vi "gxml_BldTypeAttr.vi"(4 "error out":errorcluster, 5 "Variant":variant) -> (1 "error IO":errorcluster, 2 "TypeString":string)   [LabVIEW 2011, in "Third Party VIs.lvlib" / "GXML.lvlib"]
uses:
  GXML.lvlib
  <vilib>/Utility/VariantDataType/VariantType.lvlib
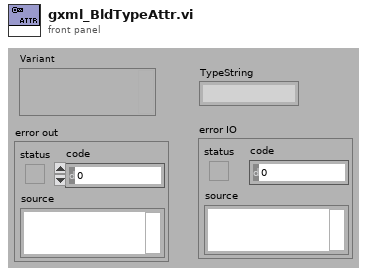
[diagram p1: front panel]
types:
  T1 = typedef "VariantType.lvlib/Type.ctl" = enum8{"Invalid Type", "Void", "I8", "I16", "I32", "I64", "U8", "U16", "U32", "U64", "Single Float", "Double Float", "Extended Float", "Single Complex", "Double Complex", "Extended Complex", "Enum U8", "Enum U16", "Enum U32", "Enum U64", "Single Float With Unit", "Double Float With Unit", "Extended Float With Unit", "Single Complex with Unit", "Double Complex with Unit", "Extended Complex with Unit", "Boolean", "String", "Path", "Picture", "Tag", "Array", "Cluster", "Variant", "LV Variant", "Waveform", "Timestamp", "Digital Waveform", "Digital Data", "ExpressData", "Refnum", "External Data", "VI", "Poly VI", "LabVIEW Class Instance", "Fixed Point"}
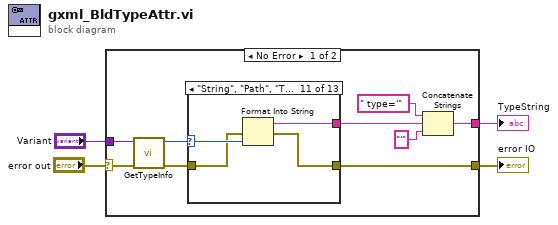
[diagram p0: block diagram]
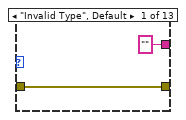
[diagram p2: hidden frame]
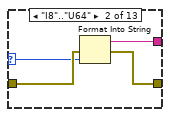
[diagram p3: hidden frame]
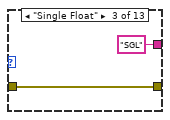
[diagram p4: hidden frame]
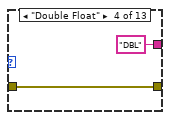
[diagram p5: hidden frame]
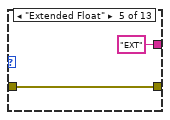
[diagram p6: hidden frame]
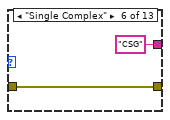
[diagram p7: hidden frame]
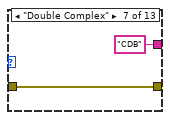
[diagram p8: hidden frame]
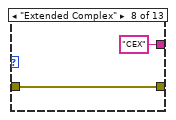
[diagram p9: hidden frame]
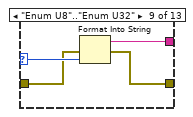
[diagram p10: hidden frame]
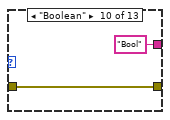
[diagram p11: hidden frame]
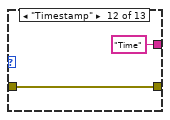
[diagram p12: hidden frame]
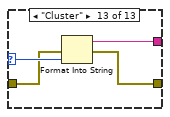
[diagram p13: hidden frame]
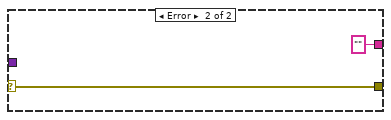
[diagram p14: hidden frame]
diagram:
  n1 = case shown="No Error" "error out" {
    selector: "error out" -> [w5 w49]
    tunnel: [w13 w49] -> w4
    tunnel: [w11 ""] -> w3
    tunnel: "Variant" -> [w7 _]
    frame No Error {
      n2 = call <vilib>:"GetTypeInfo.vi"("error in (no error)"=w5, "Variant"=w7) -> ("error out"=w8:errorcluster, "Type Enum"=w6:T1)  [unwired: 5 in, 3 out]
      n3 = case shown="\"String\", \"Path\", \"Tag\"" w6 {
        selector: w6 -> [_ w16 _ _ _ _ _ _ w35 _ w41 _ w47]
        tunnel: [w15 w19 w20 w23 w24 w26 w29 w30 w32 w37 w39 w43 w45] -> w13
        tunnel: ["" w18 "SGL" "DBL" "EXT" "CSG" "CDB" "CEX" w34 "Bool" w40 "Time" w44] -> w10
        tunnel: w8 -> [w15 w17 w20 w23 w24 w26 w29 w30 w33 w37 w38 w43 w46]
        frame "Invalid Type", Default {
        }
        frame "I8".."U64" {
          n4 = Format Into String(error in=w17, w16) -> (resulting string=w18:string, error out=w19:errorcluster)  [unwired: 2 in]
        }
        frame "Single Float" {
        }
        frame "Double Float" {
        }
        frame "Extended Float" {
        }
        frame "Single Complex" {
        }
        frame "Double Complex" {
        }
        frame "Extended Complex" {
        }
        frame "Enum U8".."Enum U32" {
          n5 = Format Into String(error in=w33, w35) -> (resulting string=w34:string, error out=w32:errorcluster)  [unwired: 2 in]
        }
        frame "Boolean" {
        }
        frame "String", "Path", "Tag" {
          n6 = Format Into String(error in=w38, w41) -> (resulting string=w40:string, error out=w39:errorcluster)  [unwired: 2 in]
        }
        frame "Timestamp" {
        }
        frame "Cluster" {
          n7 = Format Into String(error in=w46, w47) -> (resulting string=w44:string, error out=w45:errorcluster)  [unwired: 2 in]
        }
      }
      n8 = Concatenate Strings(" type='" ("string"), w10, "'" ("string")) -> (w11:string)
    }
    frame Error {
    }
  }
  "error IO" <- w4
  "TypeString" <- w3
